vi "Go To Stopping.vi"(8 "error in (no error)":errorcluster, 11 "Command.lvlib:CommandStates.lvclass 2":refnum<class "Command State.lvclass">) -> (0 "error out":errorcluster, 3 "State out":refnum<class "State Actor.lvclass">)   [LabVIEW 2013, in "Command State.lvclass"]
uses:
  Command State.lvclass
  <vilib>/ni/Actors/State Actor/State Actor/State Actor.lvclass
  Not Started/Not Started.lvclass
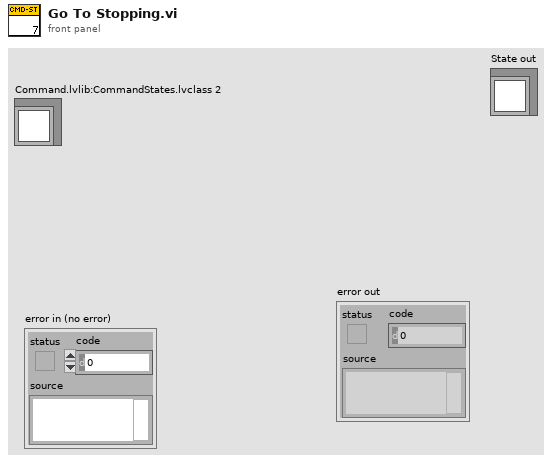
[diagram p1: front panel]
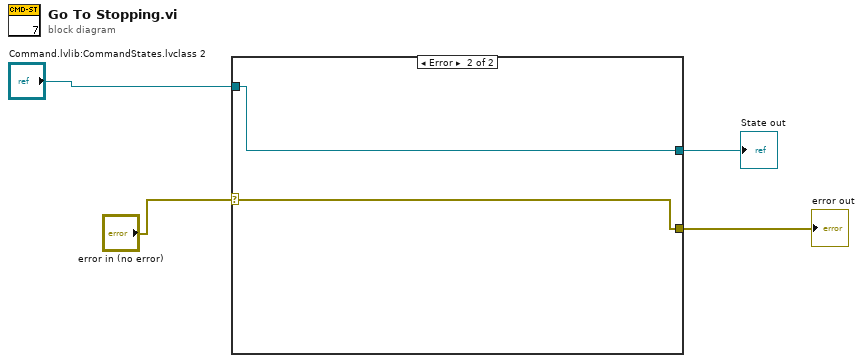
[diagram p0: block diagram]
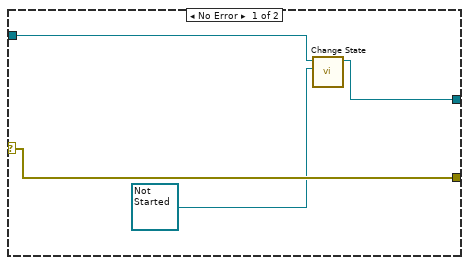
[diagram p2: hidden frame]
diagram:
  n1 = case shown="Error" "error in (no error)" {
    selector: "error in (no error)" -> [w8 w10]
    tunnel: [w8 w10] -> w3
    tunnel: [w6 w9] -> w2
    tunnel: "Command.lvlib:CommandStates.lvclass 2" -> [w5 w9]
    frame No Error {
      n2 = call <vilib>:"Change State.vi"("New State in"=refnum<class "Not Started.lvclass"> refnum ("Command.lvlib:Not Started.lvclass"), "State in"=w5) -> ("State out"=w6:refnum<class "State Actor.lvclass">)  [unwired: 8 in, 1 out]
    }
    frame Error {
    }
  }
  "error out" <- w3
  "State out" <- w2
